vi "Test Crop ARGB.vi"(8 "error in (no error)":errorcluster, 11 "Test Case In":refnum<class "Image.lvclass">) -> (0 "error out":errorcluster, 3 "Test Case Out":refnum<class "Image.lvclass">)   [LabVIEW 2020, in "g_ar_toolkit.test.lvlib" / "Image.lvclass"]
uses:
  Image.lvclass
  C:/Program Files (x86)/National Instruments/LabVIEW 2020/vi.lib/Astemes/LUnit/Test Case.lvclass
  g_ar_toolkit.common/Image Size (Integer).ctl
  <vilib>/Astemes/LUnit/Test Case.lvclass/Test Case.ctl
  g_ar_toolkit.image/CreateEmptyImageARGB.vi
  4993e8ee-a06a-463a-9684-69129f64d5ce.vi
  g_ar_toolkit.image/Copy Array to Image.vi
  g_ar_toolkit.image/CopyArrayToImageARGB.vi
  g_ar_toolkit.image/CreateEmptyImageARGB.vi/3321fa97-f432-4e1e-8db9-a0df79aed21b.vi
  g_ar_toolkit.image/CropImageARGB.vi/2dc01dea-48f6-4df4-8727-934e95e7e307.vi
  <vilib>/Astemes/LUnit/Append Pass Result.vi
  <vilib>/Astemes/LUnit/Append Fail Result.vi
  <vilib>/Astemes/LUnit/Describe Comparison.vi
  <vilib>/Astemes/LUnit/Compare Variants.vi
  g_ar_toolkit.image/CopyArrayToImageARGB.vi/26c70cee-9332-41f4-9755-08948a885cbe.vi
  <vilib>/Astemes/LUnit/Run In UI.vi
  <vilib>/Utility/error.llb/Clear Errors.vi
  g_ar_toolkit.image/ARGBColourToU32.vi
  g_ar_toolkit.common/Module Path.vi
  <vilib>/Utility/error.llb/Error Cluster From Error Code.vi
  <vilib>/picture/pixmap.llb/Flatten Pixmap.vi
  <vilib>/Astemes/LUnit/Describe Variant.vi
  Image.lvclass/Image.ctl
  g_ar_toolkit.image/g_ar_toolkit.image.lvlib
  g_ar_toolkit.common/g_ar_toolkit.common.lvlib
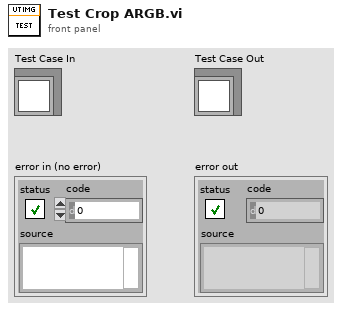
[diagram p1: front panel]
types:
  T1 = typedef "g_ar_toolkit.common.lvlib/Image Size (Integer).ctl" = cluster{"Width":u16, "Height":u16}
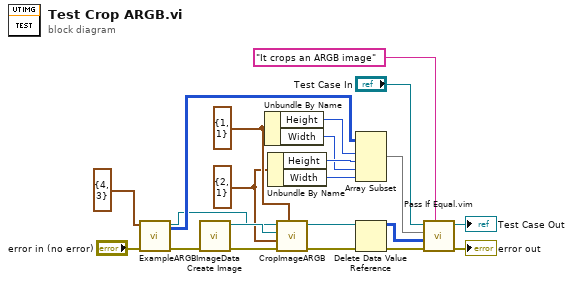
[diagram p0: block diagram]
diagram:
  w11 = T1 {"Width"=1, "Height"=1} ("Origin (Default: 0,0)")
  w10 = T1 {"Width"=2, "Height"=1} ("Cropped Size")
  n1 = call "ExampleARGBImageData.vi"("error in (no error)"="error in (no error)", "Image Size"=T1 {"Width"=4, "Height"=3}) -> ("error out"=w13:errorcluster, "Data Value Reference out"=w3:refnum<data-value>, "ARGB Array Data"=w12:u32[][])  [unwired: 6 in, 1 out]
  n2 = call-poly "Create Image.vi"("error in (no error)"=w13) -> ("error out"=w17:errorcluster, "New ARGB Image"=w15:refnum<data-value>)  [unwired: 9 in]
  n3 = Unbundle By Name(w11) -> ("Height"=w8:u16, "Width"=w7:u16)
  n4 = Unbundle By Name(w10) -> ("Height"=w9:u16, "Width"=w6:u16)
  n5 = call "CropImageARGB.vi"("Origin (Default: 0,0)"=w11, "error in (no error)"=w17, "Cropped Size"=w10, "ARGB Image Destination"=w15, "ARGB Image Source"=w3) -> ("error out"=w18:errorcluster, "ARGB Image Destination (duplicate)"=w4:refnum<data-value>)  [unwired: 5 in]
  n6 = Array Subset(array=w12, index (row)=w8, length (row)=w9, index (col)=w7, length (col)=w6) -> (w5:u32[][])
  n7 = Delete Data Value Reference(data value reference=w4, error in=w18) -> (data value=w16:u32[][], error out=w2:errorcluster)
  n8 = call "Pass If Equal.vim"("Description"="It crops an ARGB image", "error in (no error)"=w2, "Actual"=w16, "Expected"=w5, "LUnit Test Case In"="Test Case In") -> ("error out"=→"error out":errorcluster, "LUnit Test Case Out"=→"Test Case Out":refnum<class "Image.lvclass">)  [unwired: 5 in]
